vi "DigIo_example.vi"() -> ()   [LabVIEW 2012]
doc: "Equipment required: 34952 multi-function card.\n\nNOTE: This example only configures the channels. To see any real results, the user must:\n a) wire channel 006 to a DMM, either directly or through a multiplexer channel.\n b) wire an input signal into channel 5 for the totalizer to count edges.\n c) wire channel 1 output to channel 3 input to read 85 decimal for the digital input results. \n\nIn the example, the following is configured:\n\n Channel 6 of the card is configured to output a voltage of 1.234 V. \n\n Channel 5 is configured to Totalizer function, so it will count any signal input onto channel 5 and display the result. It is set to NOT clear the count when it is read.\n\n The digital IO port on channel 1 is configured to output a single byte of value 85 decimal.\n\n The digital IO port on channel 3 is configured to read a digital byte and the result is displayed."
panel:
  in  "Slot number of 34952":i16=2 min=1 max=8 step=1
  in  "VISA resource name":refnum<visa-resource-name>
  out "DIG Input Results":u32[](array[numeric]) format="%x"
  out "Totalizer Results":u32[](array[numeric])
  out "VISA/Instrument Errors":errorcluster
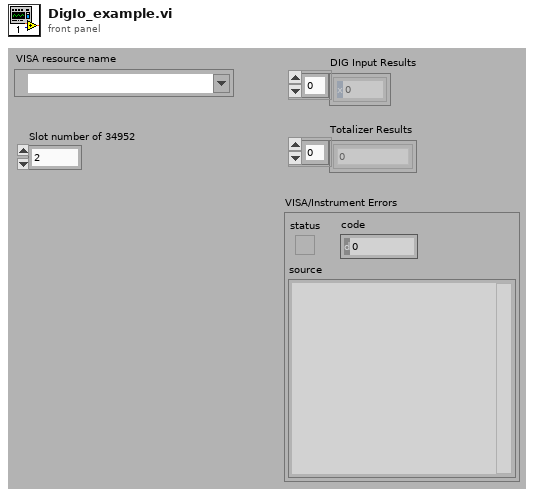
[diagram p1: front panel]
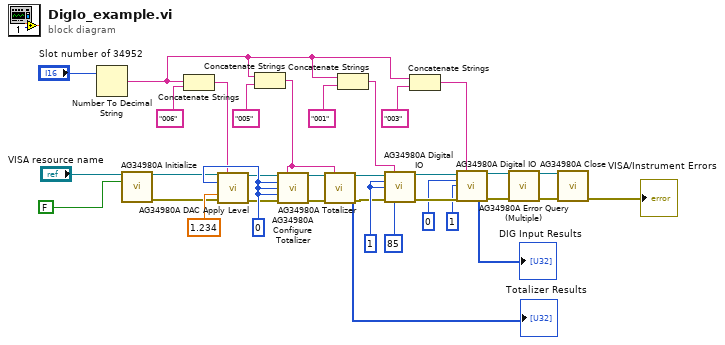
[diagram p0: block diagram]
diagram:
  w17 = 1
  w22 = 0
  n1 = Number To Decimal String(number="Slot number of 34952") -> (decimal integer string=w8:string)  [unwired: 1 in]
  n2 = call "AG34980A Initialize.vi"("VISA resource name"="VISA resource name", "ID Query (True)"=FALSE) -> ("VISA session"=w20:refnum<visa-resource-name>, "error out"=w21:errorcluster)  [unwired: 12 in]
  n3 = Concatenate Strings(w8, "006" ("string")) -> (w11:string)
  n4 = call "AG34980A DAC Apply Level.vi"("VISA resource name"=w20, "Channel List"=w11, "Source Type (0:Voltage)"=w22, "Level"=1.234, "error in (no error)"=w21) -> ("VISA resource name out"=w18:refnum<visa-resource-name>, "error out"=w19:errorcluster)  [unwired: 9 in]
  n5 = Concatenate Strings(w8, "005") -> (w10:string)
  n6 = call "AG34980A Configure Totalizer.vi"("VISA resource name"=w18, "Channel List(empty)"=w10, "Read Type (0:Read)"=w22, "Mode (0:TTL)"=w22, "Slope (0:Positive)"=w22, "error in (no error)"=w19) -> ("VISA resource name out"=w15:refnum<visa-resource-name>, "error out"=w16:errorcluster)  [unwired: 8 in]
  n7 = call "AG34980A Totalizer.vi"("VISA resource name"=w15, "Scan List"=w10, "error in (no error)"=w16) -> ("VISA resource name out"=w13:refnum<visa-resource-name>, "Output Array"=→"Totalizer Results":u32[], "error out"=w14:errorcluster)  [unwired: 10 in]
  n8 = Concatenate Strings(w8, "001") -> (w4:string)
  n9 = call "AG34980A Digital IO.vi"("VISA resource name"=w13, "Channel List"=w4, "Action (1:Write)"=w17, "Width (1:Byte)"=w17, "error in (no error)"=w14, "Data In"=85) -> ("VISA resource name out"=w33:refnum<visa-resource-name>, "error out"=w32:errorcluster)  [unwired: 7 in, 1 out]
  n10 = Concatenate Strings(w8, "003") -> (w2:string)
  n11 = call "AG34980A Digital IO.vi"("VISA resource name"=w33, "Channel List"=w2, "Action (1:Write)"=0, "Width (1:Byte)"=1, "error in (no error)"=w32) -> ("VISA resource name out"=w26:refnum<visa-resource-name>, "Data Out"=→"DIG Input Results":u32[], "error out"=w27:errorcluster)  [unwired: 8 in]
  n12 = call "AG34980A Error Query (Multiple).vi"("VISA resource name"=w26, "error in (no error)"=w27) -> ("VISA resource name out"=w25:refnum<visa-resource-name>, "error out"=w24:errorcluster)  [unwired: 10 in, 2 out]
  n13 = call "AG34980A Close.vi"("VISA resource name"=w25, "error in (no error)"=w24) -> ("error out"=→"VISA/Instrument Errors":errorcluster)  [unwired: 13 in]
